vi "MPExxx_get_arm.vi"(0 "VISA session":refnum<visa-resource-name>, 1 "error in (no error)":errorcluster) -> (2 "dup VISA session":refnum<visa-resource-name>, 3 "ARM State":string, 4 "error out":errorcluster)   [LabVIEW 2012]
doc: "This VI retrieves the state of the ARM discrete.\n\nValues:\n\n0 - ARM off\n1 - ARM on"
uses:
  MPExxx Globals.gbl
panel:
  # "MAGNA-POWER"
  # "Electronics"
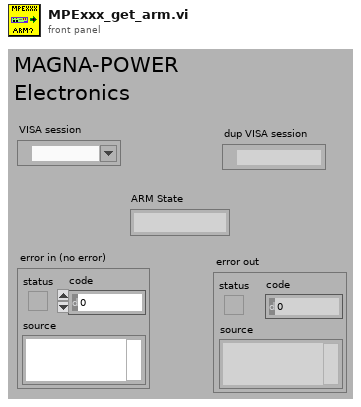
[diagram p1: front panel]
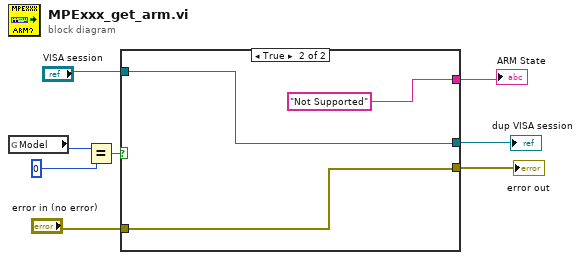
[diagram p0: block diagram]
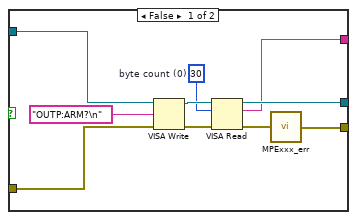
[diagram p2: hidden frame]
diagram:
  n1 = global read "MPExxx Globals.gbl" "Model"() -> (w6:u8)
  n2 = Equal?(x=w6, y=0) -> (x = y?=w8:bool)
  n3 = case shown="True" w8 {
    tunnel: "VISA session" -> [w13 w20]
    tunnel: "error in (no error)" -> [w12 w21]
    tunnel: [w11 w20] -> w3
    tunnel: [w10 w21] -> w2
    tunnel: [w9 "Not Supported"] -> w1
    frame False {
      w16 = u32 30  # byte count (0)
      n4 = VISA Write(VISA resource name=w13, write buffer="OUTP:ARM?\n", error in (no error)=w12) -> (VISA resource name out=w17:refnum<visa-resource-name>, error out=w15:errorcluster)  [unwired: 1 out]
      n5 = VISA Read(VISA resource name=w17, byte count=w16, error in (no error)=w15) -> (VISA resource name out=w11:refnum<visa-resource-name>, read buffer=w9:string, error out=w14:errorcluster)  [unwired: 1 out]
      n6 = call "MPExxx_err.vi"("error in (no error)"=w14) -> ("error out"=w10:errorcluster)
    }
    frame True {
    }
  }
  "ARM State" <- w1
  "dup VISA session" <- w3
  "error out" <- w2
